vi "UI_Monitor.vi"() -> ()   [LabVIEW 2017]
panel:
  in  "Start/Stop":bool
  in  "当前运行方向":cluster{"Down Button":bool, "Up Button":bool}
  in  "stop":bool
  out "运行指示":bool
  out "XY Graph":cluster{"X":dbl, "Y":dbl}[](graph)
  out "故障报警":bool
  in  "测试环境温度":dbl
  in  "本次运行步数":dbl
  in  "总运动步数":dbl
  in  "测量指示步位":dbl
  in  "等效运动步位":dbl
  in  "偏离零位距离":dbl
  in  "?":bool
  out "T_time":string caption="试验时间"
  out "T_Date":string caption="试验日期"
  # "低温堆棒位测量系统"
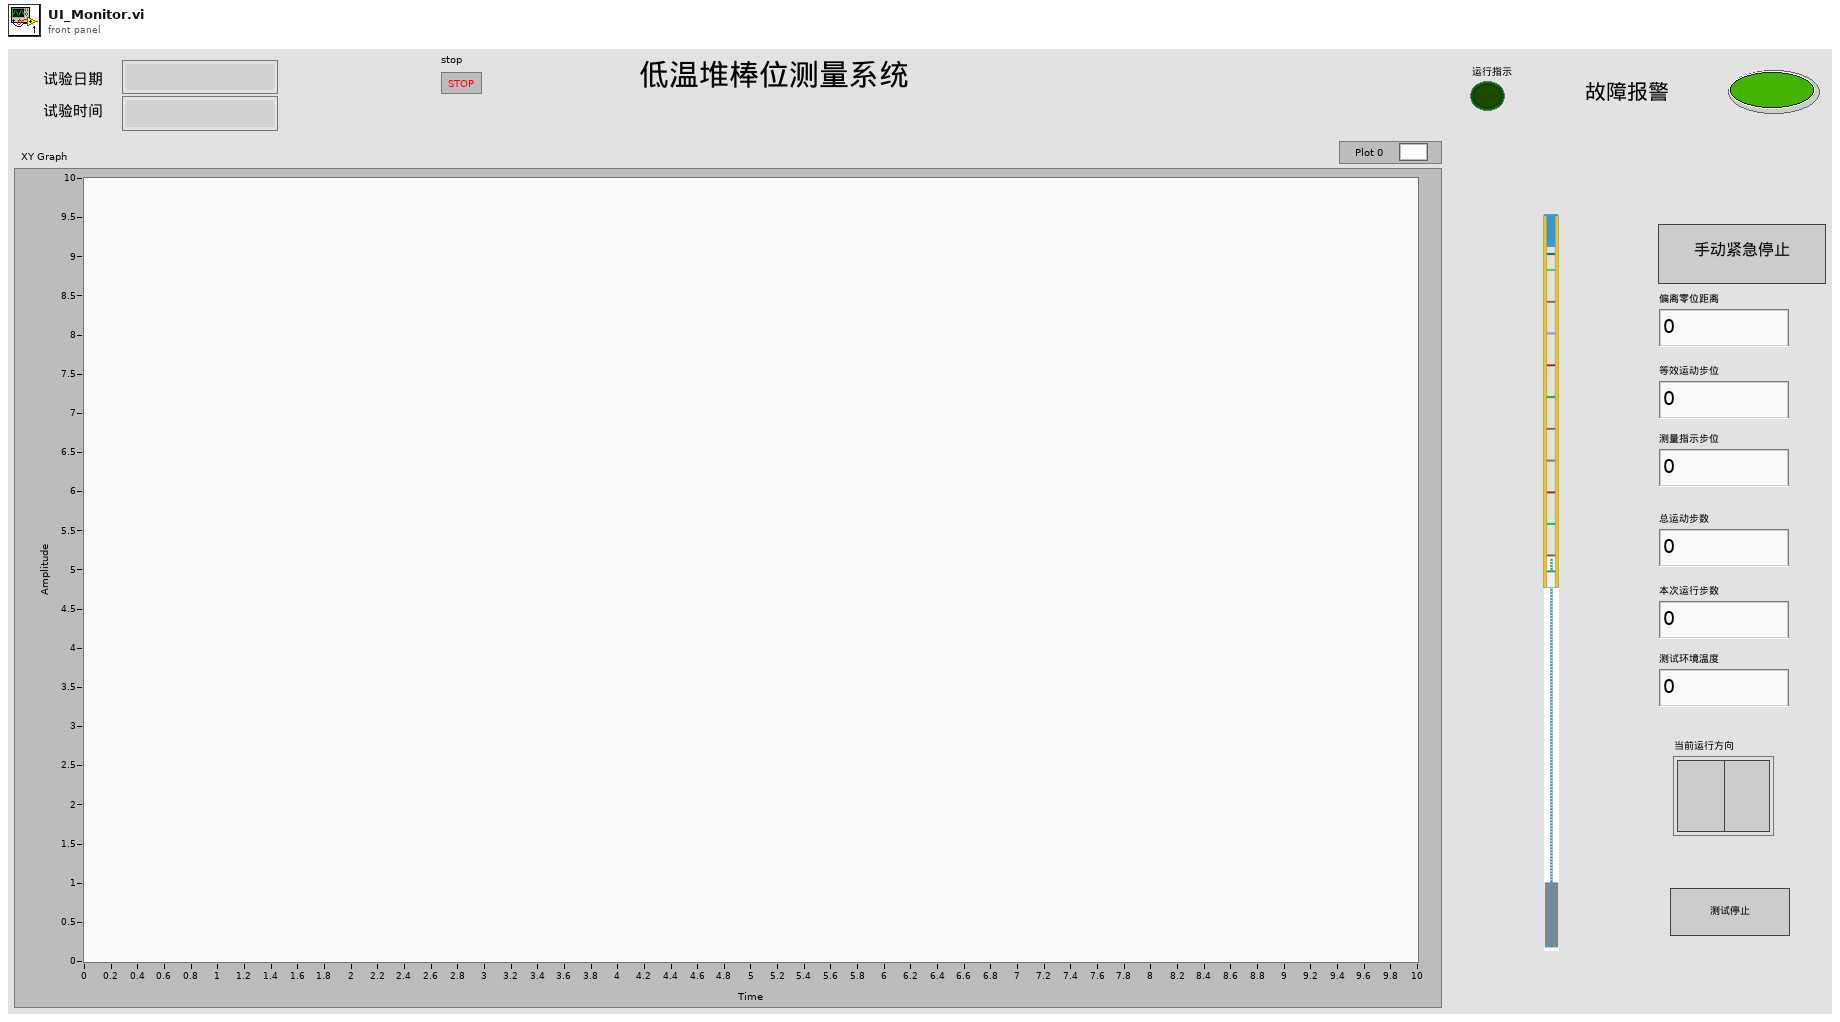
[diagram p1: front panel]
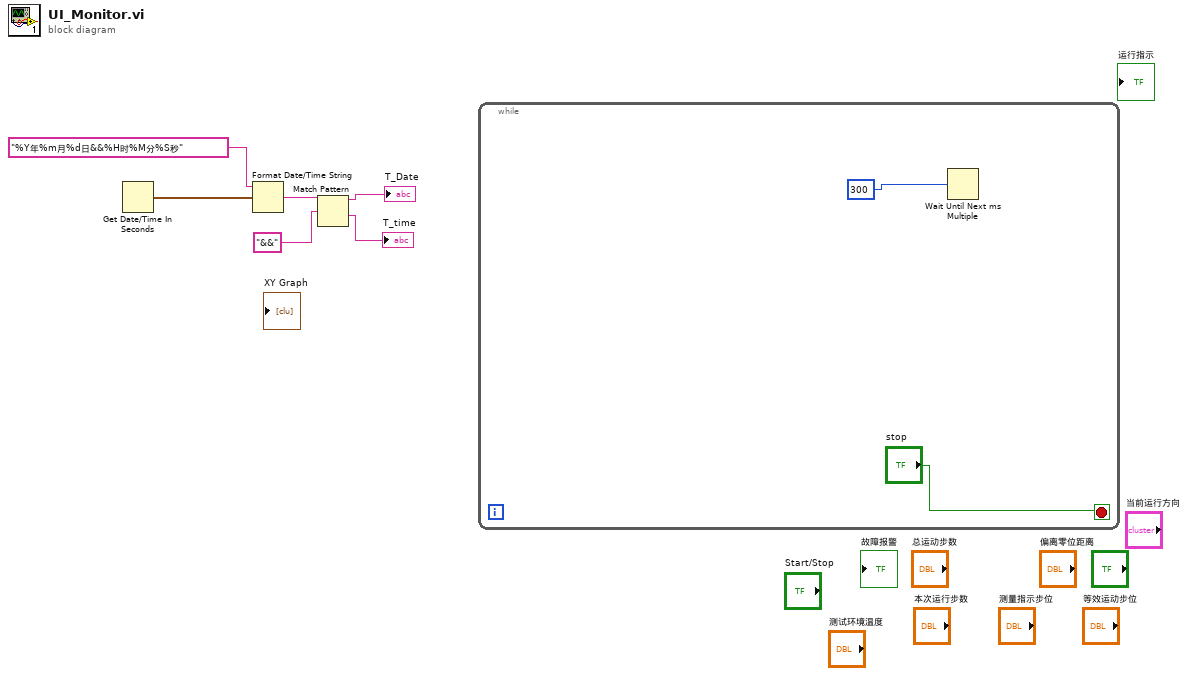
[diagram p0: block diagram]
diagram:
  n1 = Get Date/Time In Seconds() -> (seconds since 1Jan1904=w5:timestamp)
  n2 = Format Date/Time String(time format string (%c)="%Y年%m月%d日&&%H时%M分%S秒", seconds (now)=w5) -> (date/time string=w4:string)  [unwired: 1 in]
  n3 = Match Pattern(string=w4, regular expression="&&") -> (before substring=→"T_Date":string, after substring=→"T_time":string)  [unwired: 1 in, 2 out]
  n4 = while {
    stop <- "stop" stop-if-true
    n5 = Wait Until Next ms Multiple(millisecond multiple=300) -> ()  [unwired: 1 out]
  }
